vi "Get PDE Data.vi"(7 "target class":T1, 8 "error in (no error)":errorcluster, 11 "PDE in":refnum<class "NI_PDE.lvclass">) -> (0 "error out":errorcluster, 2 "PDE data":T2, 3 "PDE out":refnum<class "NI_PDE.lvclass">)   [LabVIEW 2020, in "NI_PDE.lvlib" / "NI_PDE.lvclass"]
uses:
  <vilib>/gmath/pde.llb/PDEClass/NI_PDE.lvclass
  <vilib>/gmath/pde.llb/PDEClass/PDE Data_Variant.ctl
  <vilib>/gmath/pde.llb/PDEClass/PDE Data_Class.ctl
  <vilib>/gmath/pde.llb/RHSClass/NI_RHS.lvclass
  <vilib>/gmath/pde.llb/DomainClass/NI_Domain.lvclass
  <vilib>/gmath/pde.llb/BCClass/NI_BC.lvclass
  <vilib>/gmath/pde.llb/ICClass/NI_IC.lvclass
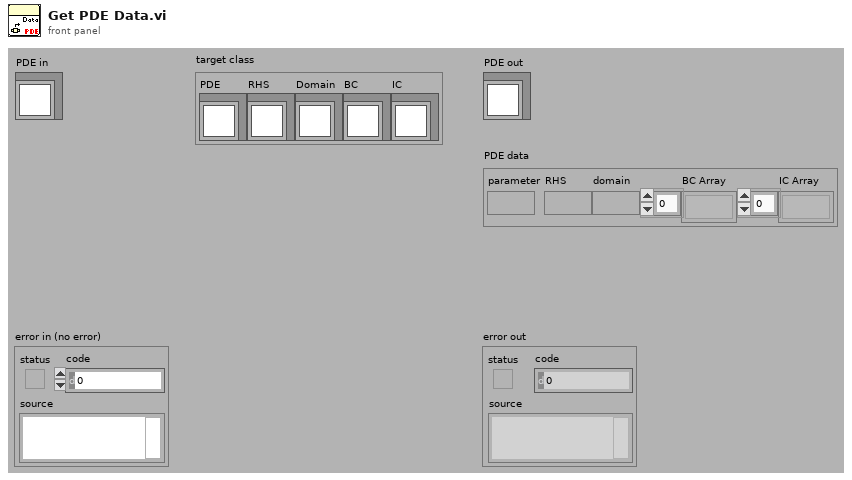
[diagram p1: front panel]
types:
  T1 = typedef "NI_PDE.lvlib/NI_PDE.lvclass/PDE Data_Class.ctl" = cluster{"PDE":refnum<class "NI_PDE.lvclass">, "RHS":refnum<class "NI_RHS.lvclass">, "Domain":refnum<class "NI_Domain.lvclass">, "BC":refnum<class "NI_BC.lvclass">, "IC":refnum<class "NI_IC.lvclass">}
  T2 = typedef "NI_PDE.lvlib/NI_PDE.lvclass/PDE Data_Variant.ctl" = cluster{"parameter":variant, "RHS":variant, "domain":variant, "BC Array":variant[], "IC Array":variant[]}
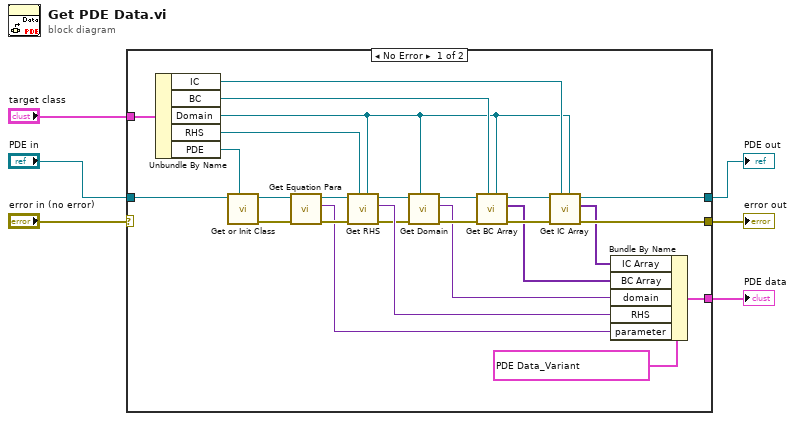
[diagram p0: block diagram]
diagram:
  n1 = case shown="No Error" "error in (no error)" {
    selector: "error in (no error)" -> [_ w33]
    tunnel: [w17 w33] -> w6
    tunnel: "PDE in" -> [w29 w34]
    tunnel: [w18 w34] -> w4
    tunnel: "target class" -> [w32 _]
    tunnel: [w31 _] -> w1
    frame No Error {
      n2 = Unbundle By Name(w32) -> ("IC"=w13:refnum<class "NI_IC.lvclass">, "BC"=w12:refnum<class "NI_BC.lvclass">, "Domain"=w10:refnum<class "NI_Domain.lvclass">, "RHS"=w11:refnum<class "NI_RHS.lvclass">, "PDE"=w9:refnum<class "NI_PDE.lvclass">)
      n3 = call <vilib>:"Get or Init Class.vi"("target PDE"=w9, "PDE in"=w29) -> ("error out"=w7:errorcluster, "PDE out"=w8:refnum<class "NI_PDE.lvclass">)  [unwired: 1 in, 7 out]
      n4 = call-dynamic "Get Equation Para.vi"("error in (no error)"=w7, "PDE in"=w8) -> ("error out"=w27:errorcluster, "parameter"=w26:variant, "PDE out"=w28:refnum<class "NI_PDE.lvclass">)  [unwired: 7 out]
      n5 = call <vilib>:"Get RHS.vi"("target Domain"=w10, "target RHS"=w11, "error in (no error)"=w27, "PDE in"=w28) -> ("error out"=w22:errorcluster, "RHS"=w25:variant, "PDE out"=w24:refnum<class "NI_PDE.lvclass">)  [unwired: 5 out]
      n6 = call <vilib>:"Get Domain.vi"("target Domain"=w10, "error in (no error)"=w22, "PDE in"=w24) -> ("error out"=w21:errorcluster, "domain"=w16:variant, "PDE out"=w23:refnum<class "NI_PDE.lvclass">)  [unwired: 6 out]
      n7 = call <vilib>:"Get BC Array.vi"("target Domain"=w10, "target BC"=w12, "error in (no error)"=w21, "PDE in"=w23) -> ("error out"=w19:errorcluster, "BC Array"=w15:variant[], "PDE out"=w20:refnum<class "NI_PDE.lvclass">)  [unwired: 1 in, 4 out]
      n8 = call <vilib>:"Get IC Array.vi"("target Domain"=w10, "target IC"=w13, "error in (no error)"=w19, "PDE in"=w20) -> ("error out"=w17:errorcluster, "IC Array"=w14:variant[], "PDE out"=w18:refnum<class "NI_PDE.lvclass">)  [unwired: 5 out]
      n9 = Bundle By Name(cluster=T2 {"parameter"=variant, "RHS"=variant, "domain"=variant, "BC Array"=[], "IC Array"=[]} ("PDE data"), "IC Array"=w14, "BC Array"=w15, "domain"=w16, "RHS"=w25, "parameter"=w26) -> (w31:T2)
    }
    frame Error {
    }
  }
  "error out" <- w6
  "PDE out" <- w4
  "PDE data" <- w1
